vi "Write Binary Message.vi"(8 "error in":errorcluster, 9 "Flattened Data":string, 10 "Message ID":u8, 11 "VISA resource in":refnum<visa-resource-name>) -> (0 "error out":errorcluster, 3 "VISA resource out":refnum<visa-resource-name>)   [LabVIEW 2019]
doc: "Builds up the binary message and then sends it through the serial port."
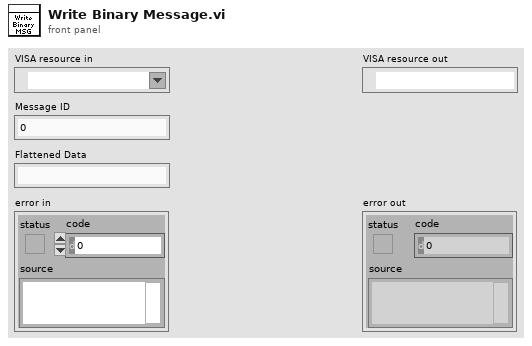
[diagram p1: front panel]
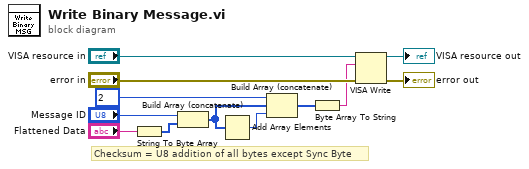
[diagram p0: block diagram]
diagram:
  # "Checksum = U8 addition of all bytes except Sync Byte"
  n1 = String To Byte Array(string="Flattened Data") -> (unsigned byte array=w8:u8[])
  n2 = Build Array (concatenate)("Message ID", w8) -> (w3:u8[])
  n3 = Add Array Elements(numeric array=w3) -> (sum=w2:u8)
  n4 = Build Array (concatenate)(u8 2 ("element"), w3, w2) -> (w1:u8[])
  n5 = Byte Array To String(unsigned byte array=w1) -> (string=w7:string)
  n6 = VISA Write(VISA resource name="VISA resource in", write buffer=w7, error in (no error)="error in") -> (VISA resource name out=→"VISA resource out":refnum<visa-resource-name>, error out=→"error out":errorcluster)  [unwired: 1 out]
